vi "Create RT FIFO.vi"   [LabVIEW 2017, in "Data Sharing Framework Engine.lvlib" / "Engine Interface.lvclass"]
uses:
  Engine Interface.lvclass
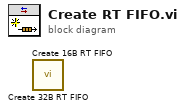
[diagram p0: block diagram]
diagram:
  n1 = call "Create 32B RT FIFO.vi"() -> ()  [unwired: 10 in, 2 out]
  n2 = call "Create 16B RT FIFO.vi"() -> ()  [unwired: 10 in, 2 out]
